vi "Process.vi"(8 "error in (no error)":errorcluster, 10 "Initialize Entry Console in":refnum<class "Initialize Entry Console.lvclass">, 11 "Architecture.lvlib:Thread.lvclass":refnum<class "Thread.lvclass">) -> (0 "error out":errorcluster, 1 "Stop?":bool, 3 "Architecture.lvlib:Thread.lvclass 2":refnum<class "Thread.lvclass">)   [LabVIEW 2013, in "Entry Console.lvlib" / "Initialize Entry Console.lvclass"]
uses:
  Initialize Entry Console.lvclass
  Thread.lvclass
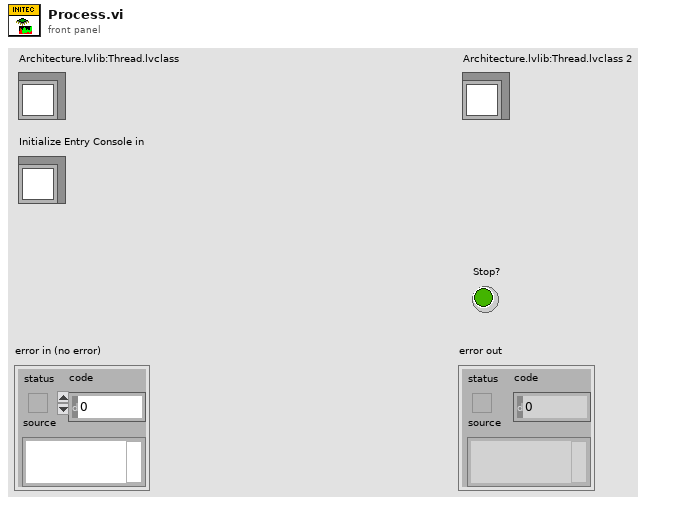
[diagram p1: front panel]
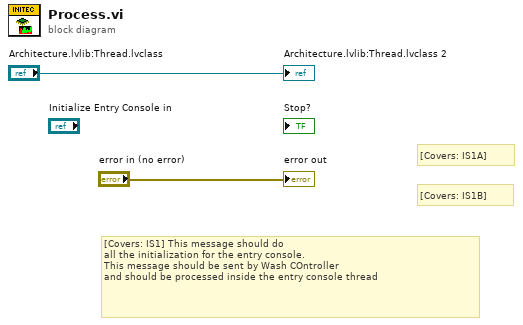
[diagram p0: block diagram]
diagram:
  # "[Covers: IS1B]"
  # "[Covers: IS1A]"
  # "[Covers: IS1] This message should do \nall the initialization for the entry console.\nThis message should be sent by Wash COntroller\nand should be processed inside the entry console thread"
  "error out" <- "error in (no error)"
  "Architecture.lvlib:Thread.lvclass 2" <- "Architecture.lvlib:Thread.lvclass"
